vi "Get DataSocket Tags.vi"(4 "All Tags":string[](array[string]), 5 "URL":string) -> (2 "DsOut":T1[](array[typedef]))   [LabVIEW 2014]
uses:
  DataSocket_Tags.ctl
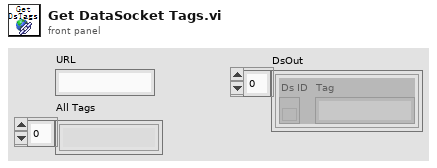
[diagram p1: front panel]
types:
  T1 = typedef "DataSocket_Tags.ctl" = cluster{"Ds ID":refnum<k13>, "Tag":string}
  T2 = enum16{"Read", "Write", "ReadWrite", "BufferedRead", "BufferedReadWrite"}
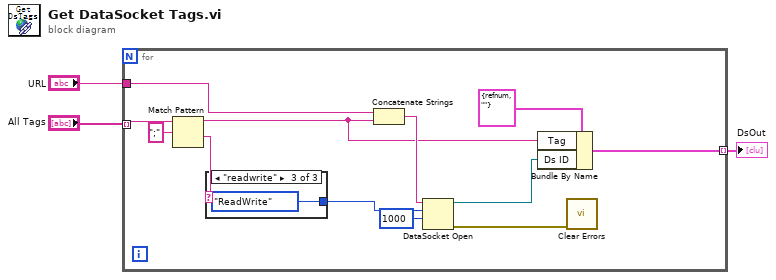
[diagram p0: block diagram]
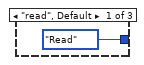
[diagram p2: hidden frame]
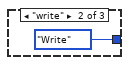
[diagram p3: hidden frame]
diagram:
  n1 = for {
    tunnel: "URL" -> [w10]
    tunnel: "All Tags" -> [w14] mode=indexing
    tunnel: [w7] -> w1 mode=indexing
    n2 = Match Pattern(string=w14, regular expression=";" ("正则表达式")) -> (before substring=w6:string, after substring=w12:string)  [unwired: 1 in, 2 out]
    n3 = case shown="\"readwrite\"" w12 {
      tunnel: [T2."Read" ("模式") T2."Write" ("模式") T2."ReadWrite" ("模式")] -> w15
      frame "read", Default {
      }
      frame "write" {
      }
      frame "readwrite" {
      }
    }
    n4 = Concatenate Strings(w10, w6) -> (w11:string)
    n5 = DataSocket Open(9:1000 ("毫秒超时(10000)"), 10:w15, 11:w11) -> (0:w5:errorcluster, 3:w8:refnum<k13>)  [unwired: 1 in]
    n6 = Bundle By Name(cluster=T1 {"Ds ID"=refnum, "Tag"=""} ("Ds Out"), "Tag"=w6, "Ds ID"=w8) -> (w7:T1)
    n7 = call <vilib>:"Clear Errors.vi"("error in (no error)"=w5) -> ()  [unwired: 5 in, 2 out]
  }
  "DsOut" <- w1
